vi "mod_NB Filter - Compensation filter design for CIC filter.vi"(2 "stop band attenuation":T1(ring)=enum."72 dB", 3 "M":i32=32) -> (0 "CIC stages":i32=9, 1 "filter coefficients":dbl[](graph))   [LabVIEW 2020, in "niAMT.lvlib"]
uses:
  <vilib>/addons/Modulation/niAMT.lvlib
  <vilib>/Analysis/1siggen.llb/Ramp Pattern by Samples.vi
  <vilib>/Analysis/NI_AALBase.lvlib
panel:
  out "h":dbl[](array[numeric]) format="%.2f"
  in  "pass band length(0..0.1)":dbl=0.013 format="%.4f"
  in  "WEIGHT":dbl=0.1 format="%.2f"
  in  "#of compensation points":i32=30
  out "error":i32
  out "ripple":dbl=1.0393984755515295e-07 format="%.2e"
  # "Decimation by two, 1/16 aliasing protection"
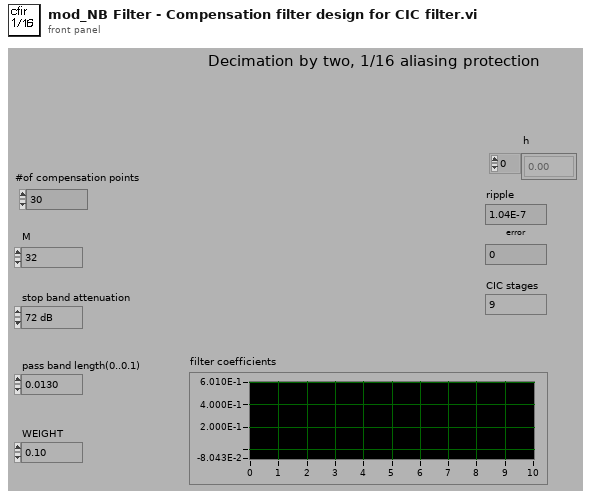
[diagram p1: front panel]
types:
  T1 = enum16{"48 dB", "60 dB", "72 dB", "84 dB", "96 dB", "120 dB"}
  T2 = cluster{"Element Data":dbl, dbl, "Element Data":dbl, "WEIGHT":dbl}[]
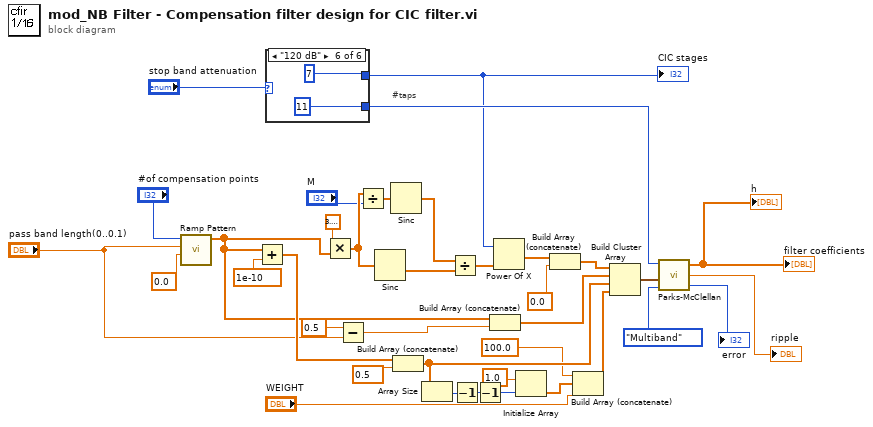
[diagram p0: block diagram]
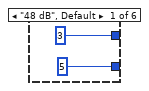
[diagram p2: hidden frame]
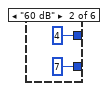
[diagram p3: hidden frame]
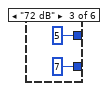
[diagram p4: hidden frame]
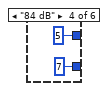
[diagram p5: hidden frame]
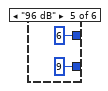
[diagram p6: hidden frame]
diagram:
  # "#taps"
  n1 = call-poly <vilib>:"Ramp Pattern.vi"("start"=0.0, "end"="pass band length(0..0.1)", "samples"="#of compensation points") -> ("Ramp Pattern"=w15:dbl[])  [unwired: 7 in, 1 out]
  n2 = Add(x=w15, y=1e-10 ("Element Data")) -> (x+y=w26:dbl[])
  n3 = case shown="\"120 dB\"" "stop band attenuation" {
    tunnel: [5 7 7 7 9 11] -> w18
    tunnel: [3 4 5 5 6 7] -> w1
    frame "48 dB", Default {
    }
    frame "60 dB" {
    }
    frame "72 dB" {
    }
    frame "84 dB" {
    }
    frame "96 dB" {
    }
    frame "120 dB" {
    }
  }
  "CIC stages" <- w1
  n4 = Multiply(x=3.141592653589793, y=w15) -> (x*y=w16:dbl[])
  n5 = Subtract(x=0.5, y="pass band length(0..0.1)") -> (x-y=w8:dbl)
  n6 = Divide(x=w16, y="M") -> (x/y=w17:dbl[])
  n7 = Sinc(1:w16) -> (0:w13:dbl[])
  n8 = Sinc(1:w17) -> (0:w14:dbl[])
  n9 = Build Array (concatenate)(w26, 0.5 ("Element Data")) -> (w23:dbl[])
  n10 = Array Size(array=w23) -> (size(s)=w32:i32)
  n11 = Divide(x=w14, y=w13) -> (x/y=w6:dbl[])
  n12 = Decrement(x=w32) -> (x-1=w11:i32)
  n13 = Decrement(x=w11) -> (x-1=w4:i32)
  n14 = Build Array (concatenate)(w15, w8) -> (w27:dbl[])
  n15 = Power Of X(1:w6, 2:w1) -> (0:w5:dbl[])
  n16 = Initialize Array(1.0 ("Element Data"), w4) -> (w30:dbl[])
  n17 = Build Array (concatenate)(w5, 0.0 ("Element Data")) -> (w34:dbl[])
  n18 = Build Array (concatenate)(100.0 ("Element Data"), w30, "WEIGHT") -> (w10:dbl[])
  n19 = Build Cluster Array(w34, w27, w23, w10) -> (w28:T2)
  n20 = call <vilib>:"Parks-McClellan.vi"("filter type"=enum32{"Multiband", "Differentiator", "Hilbert"}."Multiband", "Band Parameters"=w28, "# of taps"=w18) -> ("error"=→"error":i32, "ripple"=→"ripple":dbl, "h"=→"filter coefficients" →"h":dbl[])  [unwired: 1 in]
